vi "definitive002.vi"() -> ()   [LabVIEW 2011]
uses:
  <vilib>/DAQmx/write.llb/DAQmx Write (Digital Bool 1Line 1Point).vi
  <vilib>/DAQmx/read.llb/DAQmx Read (Analog DBL 1Chan 1Samp).vi
  <vilib>/DAQmx/create/channels.llb/DAQmx Create Channel (AI-Voltage-Basic).vi
  <vilib>/DAQmx/create/channels.llb/DAQmx Create Channel (DO-Digital Output).vi
  <vilib>/DAQmx/miscellaneous.llb/DAQmx Fill In Error Info.vi
  <vilib>/vision/NI_Vision_Development_Module.lvlib
panel:
  out "data":dbl caption="Daten" format="%0.2f"
  out "Image":T1(plugin-control)
  in  "Stop (F)":bool
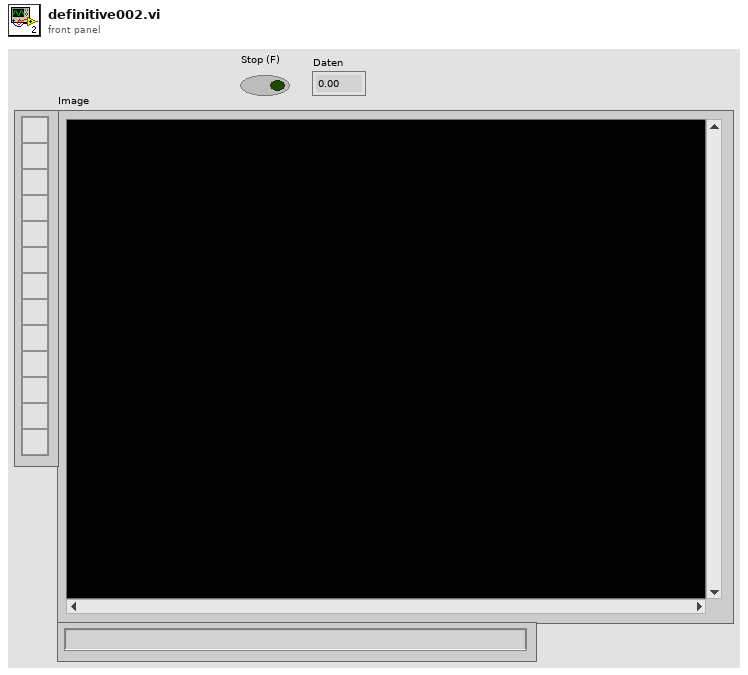
[diagram p1: front panel]
types:
  T1 = typedef "IMAQ Image.ctl" = refnum<image>
  T2 = cluster{"Position":cluster{"x":sgl, "y":sgl}, "Angle":sgl, "Scale":sgl, "Score":sgl, "Bounding Box":cluster{"x":sgl, "y":sgl}[]}[]
  T3 = cluster{"Matches (Pattern Matching 1)[0]":cluster{"Position":cluster{"x":sgl, "y":sgl}, "Angle":sgl, "Scale":sgl, "Score":sgl, "Bounding Box":cluster{"x":sgl, "y":sgl}[]}, "Matches (Pattern Matching 1)[1]":cluster{"Position":cluster{"x":sgl, "y":sgl}, "Angle":sgl, "Scale":sgl, "Score":sgl, "Bounding Box":cluster{"x":sgl, "y":sgl}[]}, "Matches (Pattern Matching 1)[2]":cluster{"Position":cluster{"x":sgl, "y":sgl}, "Angle":sgl, "Scale":sgl, "Score":sgl, "Bounding Box":cluster{"x":sgl, "y":sgl}[]}, "Matches (Pattern Matching 1)[3]":cluster{"Position":cluster{"x":sgl, "y":sgl}, "Angle":sgl, "Scale":sgl, "Score":sgl, "Bounding Box":cluster{"x":sgl, "y":sgl}[]}, "Matches (Pattern Matching 1)[4]":cluster{"Position":cluster{"x":sgl, "y":sgl}, "Angle":sgl, "Scale":sgl, "Score":sgl, "Bounding Box":cluster{"x":sgl, "y":sgl}[]}, "Matches (Pattern Matching 1)[5]":cluster{"Position":cluster{"x":sgl, "y":sgl}, "Angle":sgl, "Scale":sgl, "Score":sgl, "Bounding Box":cluster{"x":sgl, "y":sgl}[]}, "Matches (Pattern Matching 1)[6]":cluster{"Position":cluster{"x":sgl, "y":sgl}, "Angle":sgl, "Scale":sgl, "Score":sgl, "Bounding Box":cluster{"x":sgl, "y":sgl}[]}, "Matches (Pattern Matching 1)[7]":cluster{"Position":cluster{"x":sgl, "y":sgl}, "Angle":sgl, "Scale":sgl, "Score":sgl, "Bounding Box":cluster{"x":sgl, "y":sgl}[]}, "Matches (Pattern Matching 1)[8]":cluster{"Position":cluster{"x":sgl, "y":sgl}, "Angle":sgl, "Scale":sgl, "Score":sgl, "Bounding Box":cluster{"x":sgl, "y":sgl}[]}}
  T4 = cluster{"Matches (Pattern Matching 1)[0]":cluster{"Position":cluster{"x":sgl, "y":sgl}, "Angle":sgl, "Scale":sgl, "Score":sgl, "Bounding Box":cluster{"x":sgl, "y":sgl}[]}, "Matches (Pattern Matching 1)[1]":cluster{"Position":cluster{"x":sgl, "y":sgl}, "Angle":sgl, "Scale":sgl, "Score":sgl, "Bounding Box":cluster{"x":sgl, "y":sgl}[]}, "Matches (Pattern Matching 1)[2]":cluster{"Position":cluster{"x":sgl, "y":sgl}, "Angle":sgl, "Scale":sgl, "Score":sgl, "Bounding Box":cluster{"x":sgl, "y":sgl}[]}, "Matches (Pattern Matching 1)[3]":cluster{"Position":cluster{"x":sgl, "y":sgl}, "Angle":sgl, "Scale":sgl, "Score":sgl, "Bounding Box":cluster{"x":sgl, "y":sgl}[]}}
  T5 = cluster{"Bounding Box[0]":cluster{"x":sgl, "y":sgl}, "Bounding Box[1]":cluster{"x":sgl, "y":sgl}, "Bounding Box[2]":cluster{"x":sgl, "y":sgl}, "Bounding Box[3]":cluster{"x":sgl, "y":sgl}}
  T6 = cluster{"[0]":sgl, "[1]":sgl, "[2]":sgl, "[3]":sgl}
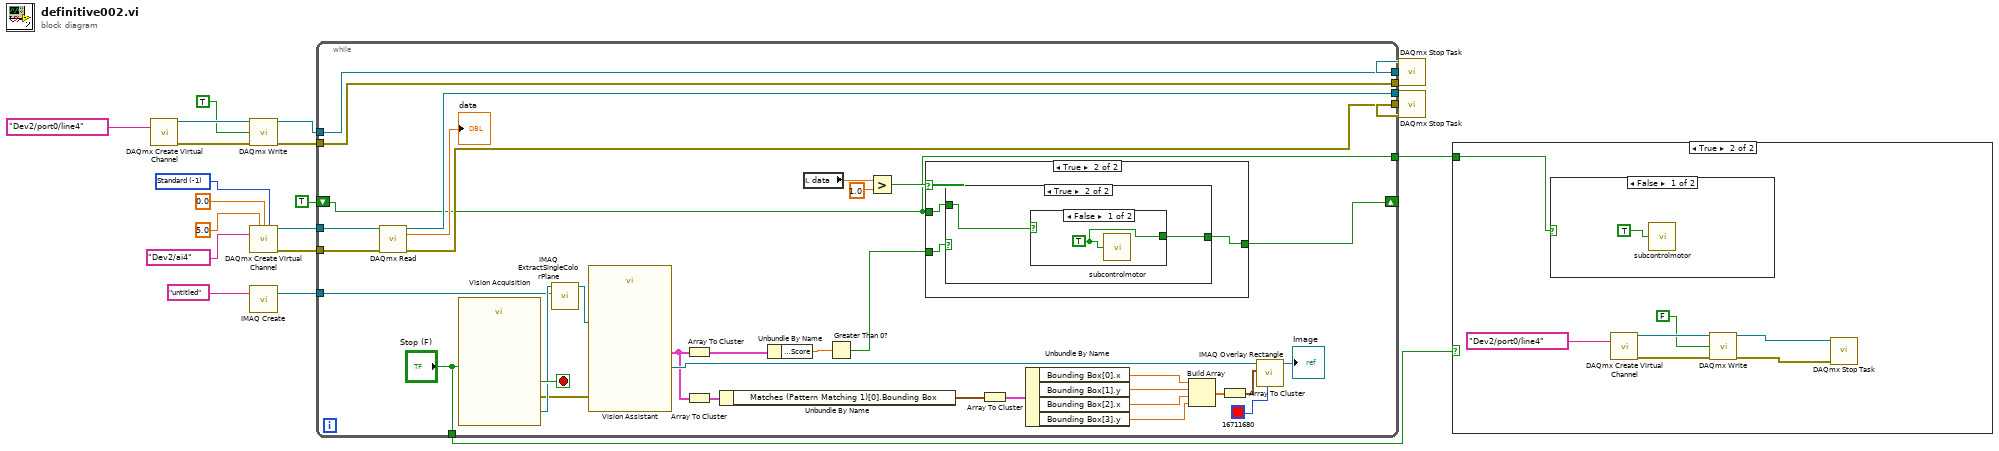
[diagram p0: block diagram]
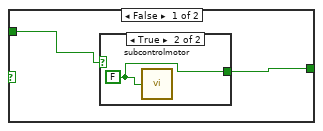
[diagram p5: hidden frame]
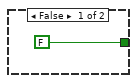
[diagram p6: hidden frame]
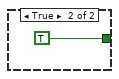
[diagram p7: hidden frame]
diagram:
  w16 = -1 items=["Standard"=-1, "RSE"=10083, "NRSE"=10078, "Differentiell"=10106, "Pseudodifferentiell"=12529] ("input terminal configuration")
  n1 = call-poly <vilib>:"DAQmx Create Virtual Channel.vi"("lines"=tag "Dev2/port0/line4") -> ("task out"=w8:refnum<k21>, "error out"=w7:errorcluster)  [unwired: 13 in]
  n2 = call-poly <vilib>:"DAQmx Write.vi"("task/channels in"=w8, "data"=TRUE, "error in"=w7) -> ("task out"=w6:refnum<k21>, "error out"=w5:errorcluster)  [unwired: 10 in, 1 out]
  n3 = call-poly <vilib>:"DAQmx Create Virtual Channel.vi"("maximum value"=5.0, "minimum value"=0.0, "input terminal configuration"=w16, "physical channels"=tag "Dev2/ai4") -> ("task out"=w15:refnum<k21>, "error out"=w14:errorcluster)  [unwired: 10 in]
  n4 = call "IMAQ Create"("Image Name"="untitled") -> ("New Image"=w20:T1)  [unwired: 4 in, 1 out]
  n5 = while {
    tunnel: w20 -> [w53]
    tunnel: w15 -> [w34]
    tunnel: w14 -> [w33]
    tunnel: [w32] -> w13
    tunnel: [w31] -> w12
    tunnel: [w29] -> w10
    tunnel: [w28] -> w9
    tunnel: w6 -> [w29]
    tunnel: w5 -> [w28]
    shift-right: [w24] -> _
    shift-left: TRUE ("Boolesch") -> [w22]
    tunnel: ["Stop (F)"] -> w2
    tunnel: [w22] -> w1
    stop <- w55 stop-if-true
    n6 = call-poly <vilib>:"DAQmx Read.vi"("task/channels in"=w34, "error in"=w33) -> ("task out"=w32:refnum<k21>, "data"=→"data":dbl, "error out"=w31:errorcluster)  [unwired: 11 in]
    n7 = call "Vision Acquisition"("Stop (F)"="Stop (F)") -> ("Image Out"=w54:T1, "Stopped"=w55:bool, "error out"=w52:errorcluster)  [unwired: 24 in]
    n8 = call "IMAQ ExtractSingleColorPlane"("Image Dst"=w53, "Image Src"=w54) -> ("Image Dst Out"=w51:T1)  [unwired: 8 in, 1 out]
    n9 = call "Vision Assistant"("Image In"=w51, "error in"=w52) -> ("Image Out"=w41:T1, "Matches (Pattern Matching 1)"=w38:T2)  [unwired: 23 in, 1 out]
    n10 = Array To Cluster(array=w38) -> (cluster=w37:T3)
    n11 = Array To Cluster(array=w38) -> (cluster=w50:T4)
    n12 = Unbundle By Name(w50) -> ("Matches (Pattern Matching 1)[0].Bounding Box"=w49:cluster{"x":sgl, "y":sgl}[])
    n13 = Unbundle By Name(w37) -> ("Matches (Pattern Matching 1)[0].Score"=w36:sgl)
    n14 = local read "data"() -> (w27:dbl)
    n15 = Greater Than 0?(x=w36) -> (x > 0?=w30:bool)
    n16 = Greater?(x=w27, y=1.0) -> (0:w25:bool)
    n17 = case shown="True" w25 {
      tunnel: w30 -> [_ w59]
      tunnel: [w56 w58] -> w24
      tunnel: w22 -> [w56 w57]
      frame False {
      }
      frame True {
        n18 = case shown="True" w59 {
          tunnel: [w61 w65] -> w58
          tunnel: w57 -> [w60 w64]
          frame False {
            n19 = case shown="True" w60 {
              tunnel: [FALSE ("Boolesch") w63] -> w61
              frame False {
              }
              frame True {
                w63 = FALSE ("Boolesch")
                n20 = call "subcontrolmotor.vi"("Boolesch"=w63) -> ()
              }
            }
          }
          frame True {
            n21 = case shown="False" w64 {
              tunnel: [w66 TRUE ("Boolesch")] -> w65
              frame False {
                w66 = TRUE ("Boolesch")
                n22 = call "subcontrolmotor.vi"("Boolesch"=w66) -> ()
              }
              frame True {
              }
            }
          }
        }
      }
    }
    n23 = Array To Cluster(array=w49) -> (cluster=w48:T5)
    n24 = Unbundle By Name(w48) -> ("Bounding Box[0].x"=w47:sgl, "Bounding Box[1].y"=w46:sgl, "Bounding Box[2].x"=w45:sgl, "Bounding Box[3].y"=w44:sgl)
    n25 = Build Array(w47, w46, w45, w44) -> (w43:sgl[])
    n26 = Array To Cluster(array=w43) -> (cluster=w42:T6)
    n27 = call "IMAQ Overlay Rectangle"("Color"=u32 16711680, "Rectangle"=w42, "Image"=w41) -> ("Image Out"=→"Image":T1)  [unwired: 7 in, 1 out]
  }
  n28 = call <vilib>:"DAQmx Stop Task.vi"("task/channels in"=w10, "error in"=w9) -> ()  [unwired: 12 in, 2 out]
  n29 = call <vilib>:"DAQmx Stop Task.vi"("task/channels in"=w13, "error in"=w12) -> ()  [unwired: 12 in, 2 out]
  n30 = case shown="True" w2 {
    tunnel: w1 -> [_ w68]
    frame False {
    }
    frame True {
      n31 = case shown="False" w68 {
        frame False {
          n32 = call "subcontrolmotor.vi"("Boolesch"=TRUE) -> ()
        }
        frame True {
        }
      }
      n33 = call-poly <vilib>:"DAQmx Create Virtual Channel.vi"("lines"=tag "Dev2/port0/line4") -> ("task out"=w73:refnum<k21>, "error out"=w72:errorcluster)  [unwired: 13 in]
      n34 = call-poly <vilib>:"DAQmx Write.vi"("task/channels in"=w73, "data"=FALSE, "error in"=w72) -> ("task out"=w70:refnum<k21>, "error out"=w69:errorcluster)  [unwired: 10 in, 1 out]
      n35 = call <vilib>:"DAQmx Stop Task.vi"("task/channels in"=w70, "error in"=w69) -> ()  [unwired: 12 in, 2 out]
    }
  }
